vi "Get-velocity-mode.vi"(8 "error in (no error)":errorcluster, 11 "Motor-Maxon in":refnum<class "Motor-Maxon.lvclass">) -> (0 "error out":errorcluster, 2 "Velocity mode":i8, 3 "Motor-Maxon out":refnum<class "Motor-Maxon.lvclass">)   [LabVIEW 2013, in "PowderDeposition.lvlib" / "Motor-Maxon.lvclass"]
uses:
  Motor-Maxon.lvclass
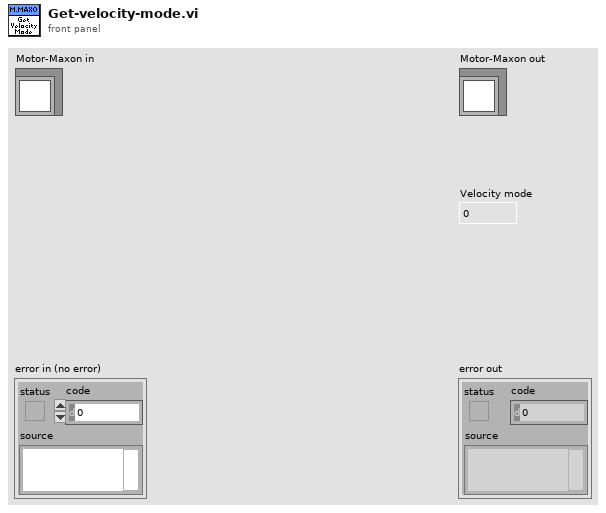
[diagram p1: front panel]
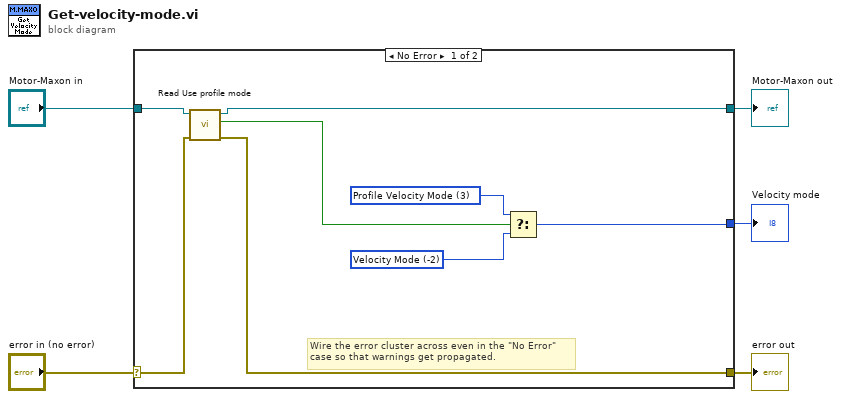
[diagram p0: block diagram]
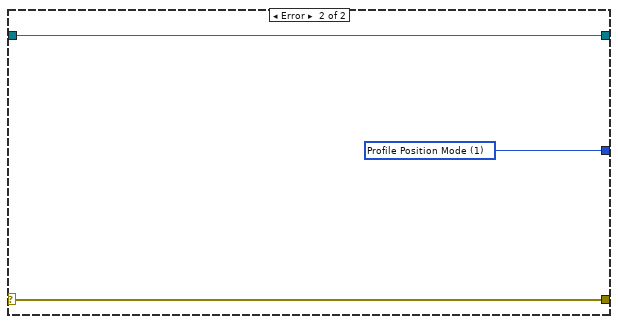
[diagram p2: hidden frame]
diagram:
  n1 = case shown="No Error" "error in (no error)" {
    selector: "error in (no error)" -> [w9 w16]
    tunnel: [w8 w16] -> w4
    tunnel: [w12 w15] -> w2
    tunnel: "Motor-Maxon in" -> [w13 w15]
    tunnel: [w6 w14] -> w1
    frame No Error {
      w7 = i8 -2 items=["Profile Position Mode"=1, "Profile Velocity Mode"=3, "Homing Mode"=6, "Interpolated Position Mode"=7, "Position Mode"=-1, "Velocity Mode"=-2, "Current Mode"=-3, "Master Encoder Mode"=-5, "Step Direction Mode"=-6] ("modes of operations")
      w11 = i8 3 items=["Profile Position Mode"=1, "Profile Velocity Mode"=3, "Homing Mode"=6, "Interpolated Position Mode"=7, "Position Mode"=-1, "Velocity Mode"=-2, "Current Mode"=-3, "Master Encoder Mode"=-5, "Step Direction Mode"=-6] ("modes of operations")
      # "Wire the error cluster across even in the \"No Error\"\ncase so that warnings get propagated."
      n2 = call-dynamic "Read Use profile mode.vi"("error in (no error)"=w9, "Motor-Maxon in"=w13) -> ("error out"=w8:errorcluster, "Use profile mode"=w10:bool, "Motor-Maxon out"=w12:refnum<class "Motor-Maxon.lvclass">)  [unwired: 7 in]
      n3 = Select(t=w11, s=w10, f=w7) -> (s? t:f=w6:i8)
    }
    frame Error {
      w14 = i8 1 items=["Profile Position Mode"=1, "Profile Velocity Mode"=3, "Homing Mode"=6, "Interpolated Position Mode"=7, "Position Mode"=-1, "Velocity Mode"=-2, "Current Mode"=-3, "Master Encoder Mode"=-5, "Step Direction Mode"=-6] ("modes of operations")
    }
  }
  "error out" <- w4
  "Motor-Maxon out" <- w2
  "Velocity mode" <- w1
